vi "Array to Cluster.vi"(5 "2D Array":string[][](array[string])) -> (2 "Address":T1(array[cluster]))   [LabVIEW 2014]
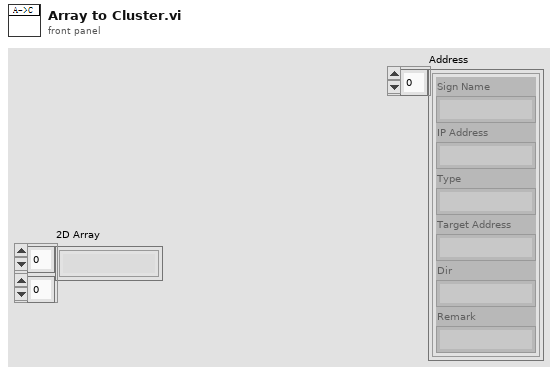
[diagram p1: front panel]
types:
  T1 = cluster{"Sign Name":string, "IP Address":string, "Type":string, "Target Address":string, "Dir":string, "Remark":string}[]
  T2 = cluster{"Sign Name":string, "English Name":string, "Type":string, "IP Address":string, "Dir":string, "Remark":string}
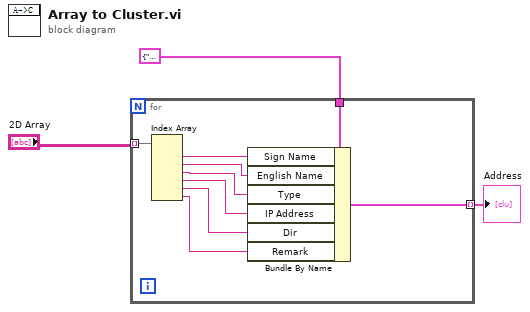
[diagram p0: block diagram]
diagram:
  n1 = for {
    tunnel: "2D Array" -> [w11] mode=indexing
    tunnel: T2 {"Sign Name"="", "English Name"="", "Type"="", "IP Address"="", "Dir"="", "Remark"=""} ("Address") -> [w12]
    tunnel: [w4] -> w1 mode=indexing
    n2 = Index Array(array=w11) -> (element #1=w10:string, element #2=w9:string, element #3=w8:string, element #4=w7:string, element #5=w6:string, element #6=w5:string)  [unwired: 6 in]
    n3 = Bundle By Name(cluster=w12, "Sign Name"=w10, "English Name"=w9, "Type"=w8, "IP Address"=w7, "Dir"=w6, "Remark"=w5) -> (w4:T2)
  }
  "Address" <- w1
